vi "manual_action-asynchronous.vi"(8 "error in (no error)":errorcluster, 10 "data":variant, 11 "step":string) -> (0 "error out":errorcluster)   [LabVIEW 2015, in "lv-recipe-machine.lvlib"]
uses:
  lv-recipe-machine.lvlib
  _controls/error.ctl
  _controls/manual_state.ctl
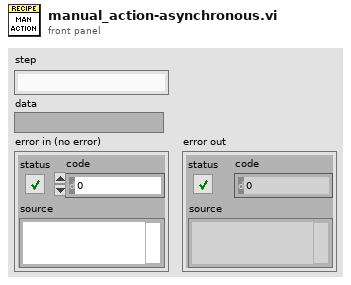
[diagram p1: front panel]
types:
  T1 = typedef "lv-recipe-machine.lvlib/error.ctl" = enum16{"<error>", "bad_command", "command_queue_timeout", "stop_notifier_timeout", "die_command_timeout", "not_in_manual_mode", "not_in_automatic_mode", "not_in_automatic_idle", "not_in_automatic_running", "not_in_automatic_paused", "automatic_step_not_found", "manual_action_not_found", "automatic_not_transition_vi", "transition_step_not_found", "unsupported_vi_type", "<null>"}
  T2 = typedef "lv-recipe-machine.lvlib/manual_state.ctl" = enum16{"<manual_state>", "failed", "action", "running", "idle", "<null>"}
  T3 = typedef "lv-recipe-machine.lvlib/references.ctl" = cluster{"semaphore":T4, "input_queue":refnum<queue>, "output_queue":refnum<queue>, "transition_queue":refnum<queue>, "data_dvr":refnum<data-value>, "stop_notifier":refnum<notifier>, "change_in_event":refnum<user-event>, "change_out_event":refnum<user-event>, "status_event":refnum<user-event>}
  T4 = typedef "Semaphore RefNum" = refnum<k1>
  T5 = typedef "lv-recipe-machine.lvlib/data.ctl" = cluster{"configuration":T6, "working":cluster{"recipe_data":T7}}
  T6 = typedef "lv-recipe-machine.lvlib/configuration.ctl" = cluster{"change_in_timeout_ms":i32}
  T7 = typedef "lv-recipe-machine.lvlib/recipe_data.ctl" = cluster{"mode":T8, "manual_state":T2, "automatic_state":T9, "previous_automatic_state":T9, "error":errorcluster, "timer []":T10[], "manual":cluster{"step_action":string, "data":variant, "actions":variant}, "automatic":cluster{"data":variant, "steps":variant, "criteria":variant, "transition":string, "index":i32, "step_launched":bool, "recipe []":T11[]}}
  T8 = typedef "lv-recipe-machine.lvlib/mode.ctl" = enum16{"<mode>", "manual", "automatic", "<null>"}
  T9 = typedef "lv-recipe-machine.lvlib/automatic_state.ctl" = enum16{"<automatic_state>", "failed", "idle", "running", "paused", "stopped", "<null>"}
  T10 = typedef "lv-recipe-machine.lvlib/timer.ctl" = cluster{"elapsed_time":dbl, "previous_time":dbl}
  T11 = typedef "lv-recipe-machine.lvlib/recipe_step.ctl" = cluster{"step":string, "data":variant}
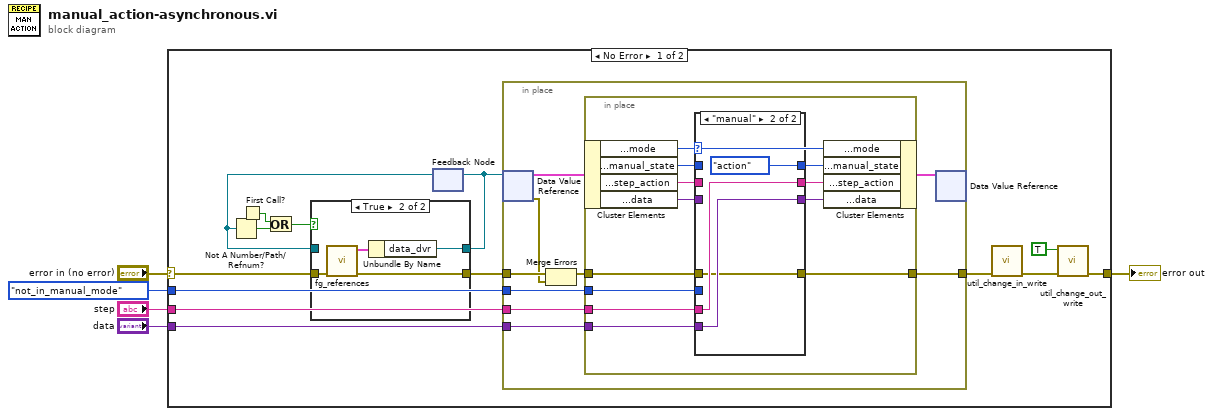
[diagram p0: block diagram]
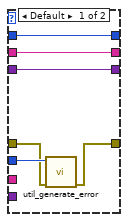
[diagram p3: hidden frame]
diagram:
  n1 = case shown="No Error" "error in (no error)" {
    selector: "error in (no error)" -> [w6 w57]
    tunnel: [w17 w57] -> w4
    tunnel: "step" -> [w19 _]
    tunnel: "data" -> [w16 _]
    tunnel: error."not_in_manual_mode" ("error") -> [w14 _]
    frame No Error {
      n2 = First Call?() -> (First Call?: T/F=w11:bool)
      n3 = feedback #1() -> (w10:refnum<data-value>)  [unwired: 1 in]
      n4 = Not A Number/Path/Refnum?(number/path/refnum=w10) -> (NaN/Path/Refnum?=w12:bool)
      n5 = Or(x=w11, y=w12) -> (x .or. y?=w9:bool)
      n6 = case shown="True" w9 {
        tunnel: w6 -> [w20 w25]
        tunnel: [w20 w24] -> w7
        tunnel: [w21 w22] -> w8
        tunnel: w10 -> [w21 _]
        frame False {
        }
        frame True {
          n7 = call "fg_references.vi"("error in (no error)"=w25) -> ("error out"=w24:errorcluster, "references out"=w23:T3)  [unwired: 9 in]
          n8 = Unbundle By Name(w23) -> ("data_dvr"=w22:refnum<data-value>)
        }
      }
      n9 = feedback-in #1(w8) -> ()
      n10 = in-place {
        in-place-border: w7 -> [w34]
        in-place-border: w19 -> [w32]
        in-place-border: w16 -> [w31]
        in-place-border: [w27] -> w15
        in-place-border: w14 -> [w26]
        n11 = in-place-dvr #2(w8) -> (w30:T5, w33:errorcluster)
        n12 = Merge Errors(w34, w33) -> (w28:errorcluster)
        n13 = in-place {
          in-place-border: w32 -> [w44]
          in-place-border: w31 -> [w45]
          in-place-border: w28 -> [w46]
          in-place-border: [w36] -> w27
          in-place-border: w26 -> [w35]
          n14 = in-place-cluster #3(w30) -> ("working.recipe_data.mode"=w41:T8, "working.recipe_data.manual_state"=w43:T2, "working.recipe_data.manual.step_action"=w40:string, "working.recipe_data.manual.data"=w39:variant)
          n15 = case shown="\"manual\"" w41 {
            tunnel: w46 -> [w48 w53]
            tunnel: w45 -> [_ w54]
            tunnel: w44 -> [_ w55]
            tunnel: w43 -> [w52 _]
            tunnel: [w52 manual_state."action" ("manual_state")] -> w42
            tunnel: w40 -> [w51 _]
            tunnel: w39 -> [w50 _]
            tunnel: [w51 w55] -> w38
            tunnel: [w50 w54] -> w37
            tunnel: [w47 w53] -> w36
            tunnel: w35 -> [w49 _]
            frame Default {
              n16 = call "util_generate_error.vi"("error in (no error)"=w48, "error"=w49) -> ("error out"=w47:errorcluster)  [unwired: 9 in]
            }
            frame "manual" {
            }
          }
          n17 = in-place-cluster #3("working.recipe_data.mode"=w41, "working.recipe_data.manual_state"=w42, "working.recipe_data.manual.step_action"=w38, "working.recipe_data.manual.data"=w37) -> (w29:T5)
        }
        n18 = in-place-dvr #2(w29) -> ()  [unwired: 2 out]
      }
      n19 = call "util_change_in_write.vi"("error in (no error)"=w15) -> ("error out"=w18:errorcluster)  [unwired: 10 in]
      n20 = call "util_change_out_write.vi"("error in (no error)"=w18, "change"=TRUE) -> ("error out"=w17:errorcluster)  [unwired: 9 in]
    }
    frame Error {
    }
  }
  "error out" <- w4
